vi "Insert LVtype into Object.vi"(5 "Item Name":string, 6 "Object (or Item) Path":string, 7 "error in (no error)":errorcluster, 8 "Value to Insert":variant, 9 "Object Offset":i32, 10 "JSON in":string="{}") -> (0 "error out":errorcluster, 1 "Replaced":bool, 3 "<JSON>":string)   [LabVIEW 2015, in "JSONtext.lvlib"]
doc: "Insert a LabVIEW Value, converted to JSON, at the Path specified."
uses:
  JSONtext.lvlib
  Variant to JSON Text.vi
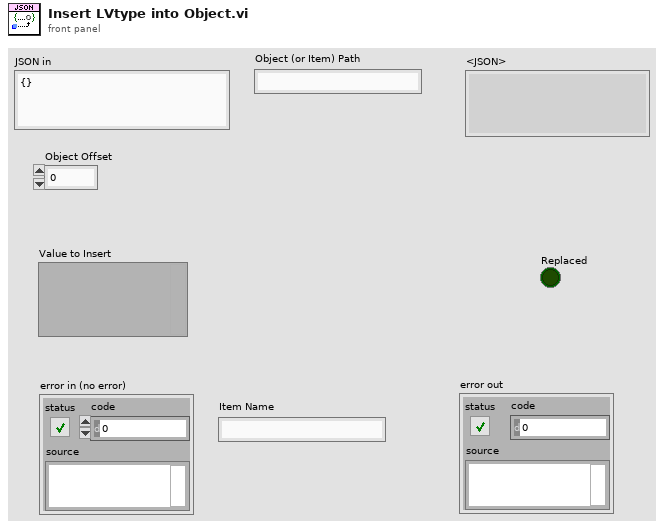
[diagram p1: front panel]
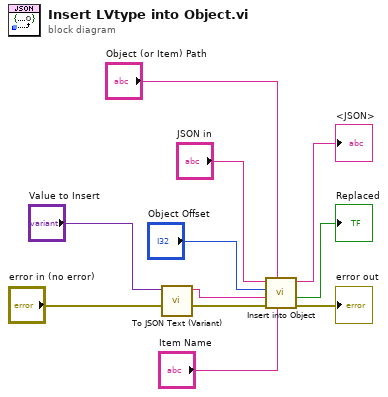
[diagram p0: block diagram]
diagram:
  n1 = call "To JSON Text (Variant).vi"("error in (no error)"="error in (no error)", "Variant"="Value to Insert") -> ("error out"=w8:errorcluster, "<JSON>"=w1:string)  [unwired: 8 in]
  n2 = call "Insert into Object.vi"("Item Name"="Item Name", "Object (or Item) Path"="Object (or Item) Path", "error in (no error)"=w8, "JSON to Insert"=w1, "Object Offset"="Object Offset", "JSON in"="JSON in") -> ("error out"=→"error out":errorcluster, "Replaced"=→"Replaced":bool, "<JSON>"=→"<JSON>":string)  [unwired: 2 in]
